vi "Main_11a.vi"() -> ()   [LabVIEW 2020]
uses:
  4985a7b0-beb7-44e5-b21a-1b7cc2dea417.vi
  <vilib>/Comparison/Less/Less Functor/Less Functor.lvclass
panel:
  out "Post Round":T1(array[cluster])
  out "Answer":i32
  in  "Puzzle":string="Monkey 0:\n  Starting items: 72, 97\n  Operation: new = old * 13\n  Test: divisible by 19\n    If true: throw to monkey 5\n    If false: throw to monkey 6\n\nMonkey 1:\n  Starting items: 55, 70, 90, 74, 95\n  Operation: new = old * old\n  Test: divisible by 7\n    If true: throw to monkey 5\n    If false: throw to monkey 0\n\nMonkey 2:\n  Starting items: 74, 97, 66, 57\n  Operation: new = old + 6\n  Test: divisible by 17\n    If true: throw to monkey 1\n    If false: throw to monkey 0\n\nMonkey 3:\n  Starting items: 86, 54, 53\n  Operation: new = old + 2\n  Test: divisible by 13\n    If true: throw to monkey 1\n    If false: throw to monkey 2\n\nMonkey 4:\n  Starting items: 50, 65, 78, 50, 62, 99\n  Operation: new = old + 3\n  Test: divisible by 11\n    If true: throw to monkey 3\n    If false: throw to monkey 7\n\nMonkey 5:\n  Starting items: 90\n  Operation: new = old + 4\n  Test: divisible by 2\n    If true: throw to monkey 4\n    If false: throw to monkey 6\n\nMonkey 6:\n  Starting items: 88, 92, 63, 94, 96, 82, 53, 53\n  Operation: new = old + 8\n  Test: divisible by 5\n    If true: throw to monkey 4\n    If false: throw to monkey 7\n\nMonkey 7:\n  Starting items: 70, 60, 71, 69, 77, 70, 98\n  Operation: new = old * 7\n  Test: divisible by 3\n    If true: throw to monkey 2\n    If false: throw to monkey 3"
  in  "Example":string="Monkey 0:\n  Starting items: 79, 98\n  Operation: new = old * 19\n  Test: divisible by 23\n    If true: throw to monkey 2\n    If false: throw to monkey 3\n\nMonkey 1:\n  Starting items: 54, 65, 75, 74\n  Operation: new = old + 6\n  Test: divisible by 19\n    If true: throw to monkey 2\n    If false: throw to monkey 0\n\nMonkey 2:\n  Starting items: 79, 60, 97\n  Operation: new = old * old\n  Test: divisible by 13\n    If true: throw to monkey 1\n    If false: throw to monkey 3\n\nMonkey 3:\n  Starting items: 74\n  Operation: new = old + 3\n  Test: divisible by 17\n    If true: throw to monkey 0\n    If false: throw to monkey 1"
  # "58056"
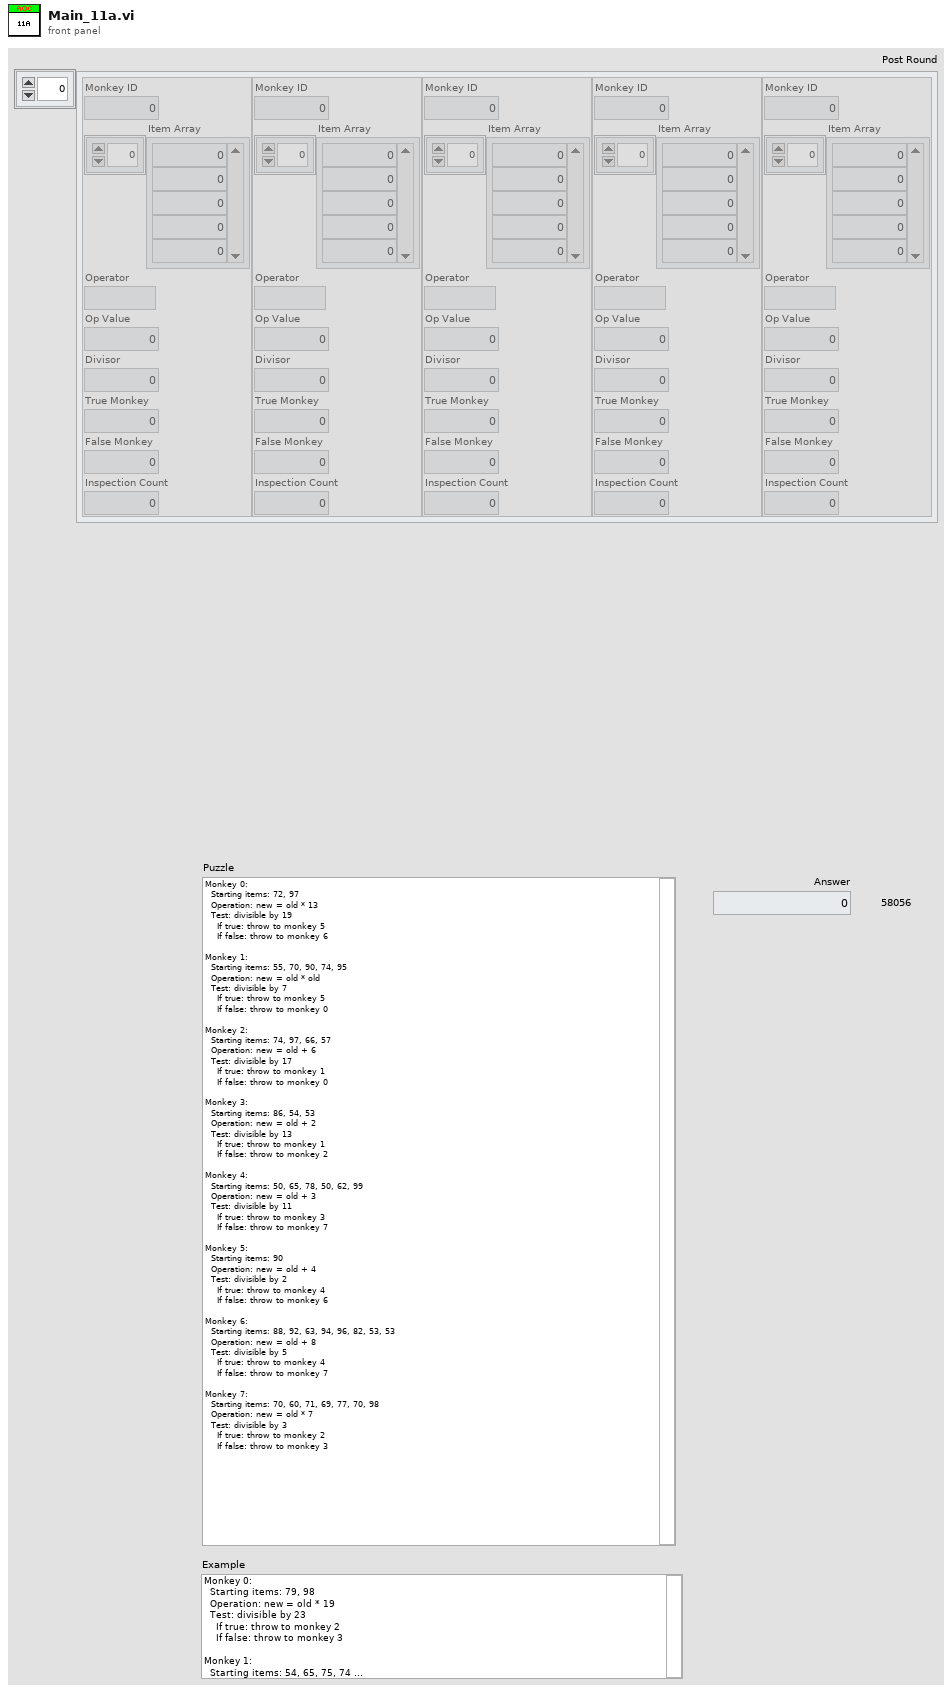
[diagram p1: front panel]
types:
  T1 = cluster{"Monkey ID":i32, "Item Array":i32[], "Operator":string, "Op Value":i32, "Divisor":i32, "True Monkey":i32, "False Monkey":i32, "Inspection Count":i32}[]
  T2 = cluster{"Monkey ID":i32, "Item Array":i32[], "Operator":string, "Op Value":i32, "Divisor":i32, "True Monkey":i32, "False Monkey":i32, "Inspection Count":i32}
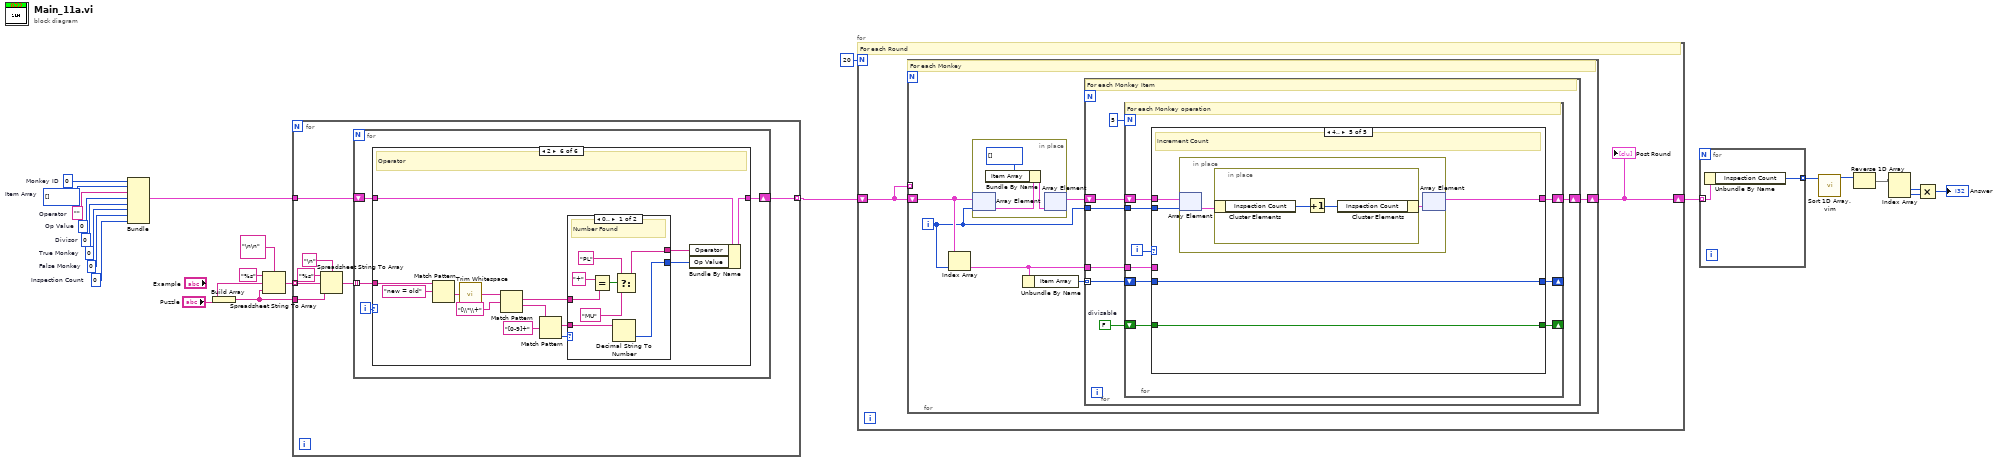
[diagram p0: block diagram]
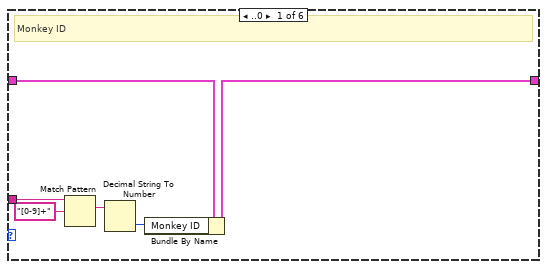
[diagram p2: hidden frame]
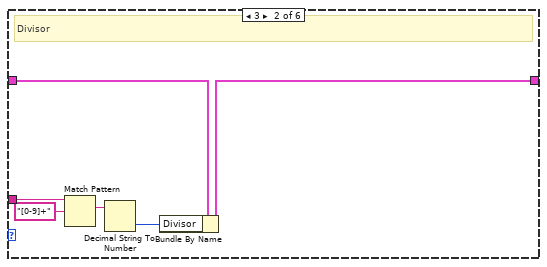
[diagram p3: hidden frame]
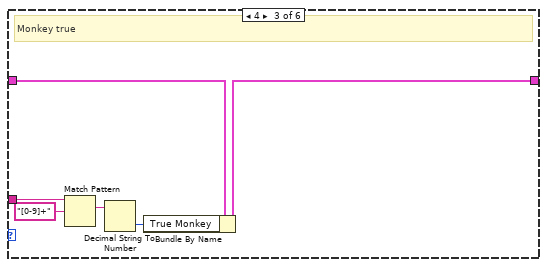
[diagram p4: hidden frame]
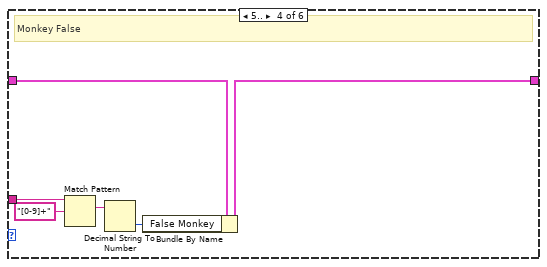
[diagram p5: hidden frame]
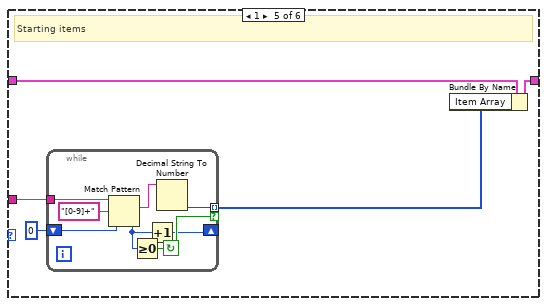
[diagram p6: hidden frame]
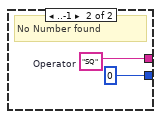
[diagram p7: hidden frame]
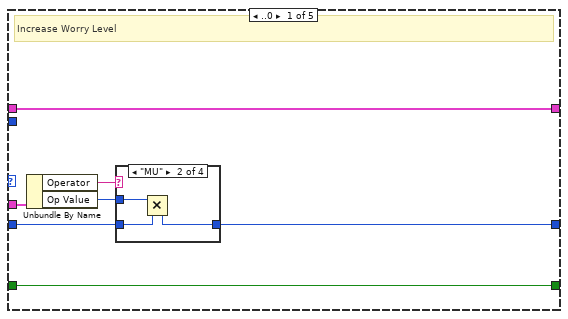
[diagram p8: hidden frame]
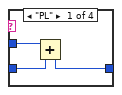
[diagram p9: hidden frame]
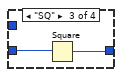
[diagram p10: hidden frame]
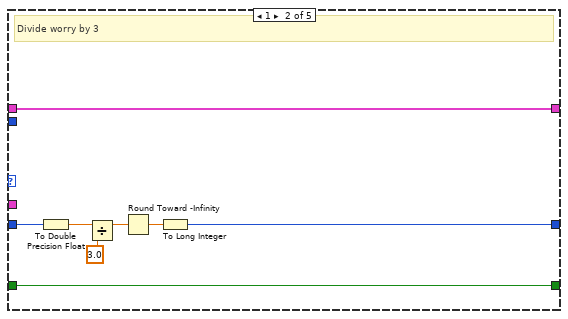
[diagram p12: hidden frame]
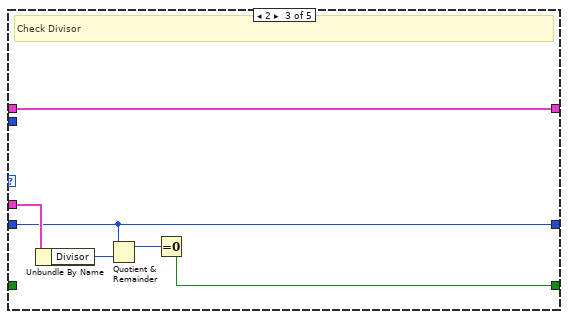
[diagram p13: hidden frame]
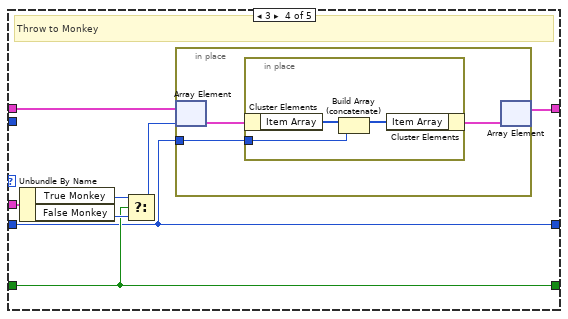
[diagram p14: hidden frame]
diagram:
  w9 = 0  # Inspection Count
  w12 = 0  # False Monkey
  w13 = 0  # True Monkey
  w14 = 0  # Divisor
  w15 = 0  # Op Value
  w16 = ""  # Operator
  w17 = i32[] []  # Item Array
  w18 = 0  # Monkey ID
  n1 = Bundle("Monkey ID"=w18, "Item Array"=w17, "Operator"=w16, "Op Value"=w15, "Divisor"=w14, "True Monkey"=w13, "False Monkey"=w12, "Inspection Count"=w9) -> (w11:T2)  [unwired: 1 in]
  n2 = Build Array("Puzzle") -> (w19:string[])
  n3 = Spreadsheet String To Array(delimiter (Tab)="\n\n", format string="%s", spreadsheet string="Puzzle", array type (2D Dbl)=w19) -> (array=w20:string[])
  n4 = for {
    tunnel: w20 -> [w30] mode=indexing
    tunnel: w19 -> [w27]
    tunnel: w11 -> [w25]
    tunnel: [w24] -> w10 mode=indexing
    n5 = Spreadsheet String To Array(delimiter (Tab)="\n", format string="%s", spreadsheet string=w30, array type (2D Dbl)=w27) -> (array=w26:string[])
    n6 = for {
      tunnel: w26 -> [w31] mode=indexing
      shift-right: [w32] -> w24
      shift-left: w25 -> [w33]
      i -> [w34]
      n7 = case shown="2" w34 {
        tunnel: w33 -> [w40 w46 w52 w58 w63 w85]
        tunnel: [w39 w45 w51 w57 w62 w84] -> w32
        tunnel: w31 -> [w38 w44 w50 w56 w61 w83]
        frame ..0 {
          # "Monkey ID"
          n8 = Match Pattern(string=w38, regular expression="[0-9]+") -> (match substring=w36:string)  [unwired: 1 in, 3 out]
          n9 = Decimal String To Number(string=w36) -> (number=w35:i32)  [unwired: 2 in, 1 out]
          n10 = Bundle By Name(cluster=w40, "Monkey ID"=w35) -> (w39:T2)
        }
        frame 3 {
          # "Divisor"
          n11 = Match Pattern(string=w44, regular expression="[0-9]+") -> (match substring=w42:string)  [unwired: 1 in, 3 out]
          n12 = Decimal String To Number(string=w42) -> (number=w41:i32)  [unwired: 2 in, 1 out]
          n13 = Bundle By Name(cluster=w46, "Divisor"=w41) -> (w45:T2)
        }
        frame 4 {
          # "Monkey true"
          n14 = Match Pattern(string=w50, regular expression="[0-9]+") -> (match substring=w48:string)  [unwired: 1 in, 3 out]
          n15 = Decimal String To Number(string=w48) -> (number=w47:i32)  [unwired: 2 in, 1 out]
          n16 = Bundle By Name(cluster=w52, "True Monkey"=w47) -> (w51:T2)
        }
        frame 5.. {
          # "Monkey False"
          n17 = Match Pattern(string=w56, regular expression="[0-9]+") -> (match substring=w54:string)  [unwired: 1 in, 3 out]
          n18 = Decimal String To Number(string=w54) -> (number=w53:i32)  [unwired: 2 in, 1 out]
          n19 = Bundle By Name(cluster=w58, "False Monkey"=w53) -> (w57:T2)
        }
        frame 1 {
          # "Starting items"
          n20 = while {
            tunnel: w61 -> [w71]
            tunnel: [w67] -> w60 mode=indexing if=w69
            shift-right: [w65] -> _
            shift-left: 0 -> [w64]
            stop <- w69 continue-if-true
            n21 = Match Pattern(string=w71, regular expression="[0-9]+", offset (0)=w64) -> (match substring=w68:string, offset past match=w66:i32)  [unwired: 2 out]
            n22 = Greater Or Equal To 0?(x=w66) -> (x >= 0?=w69:bool)
            n23 = Increment(x=w66) -> (x+1=w65:i32)
            n24 = Decimal String To Number(string=w68) -> (number=w67:i32)  [unwired: 2 in, 1 out]
          }
          n25 = Bundle By Name(cluster=w63, "Item Array"=w60) -> (w62:T2)
        }
        frame 2 {
          # "Operator"
          n26 = Match Pattern(string=w83, regular expression="new = old") -> (after substring=w81:string)  [unwired: 1 in, 3 out]
          n27 = call <vilib>:"Trim Whitespace.vi"("string"=w81) -> ("trimmed string"=w79:string)  [unwired: 1 in]
          n28 = Match Pattern(string=w79, regular expression="[\\*\\+") -> (match substring=w73:string, after substring=w78:string)  [unwired: 1 in, 2 out]
          n29 = Match Pattern(string=w78, regular expression="[0-9]+") -> (match substring=w72:string, offset past match=w76:i32)  [unwired: 1 in, 2 out]
          n30 = case shown="0.." w76 {
            tunnel: [w88 w95] -> w75
            tunnel: [w86 0] -> w74
            tunnel: w73 -> [w92 _]
            tunnel: w72 -> [w87 _]
            frame 0.. {
              # "Number Found"
              n31 = Equal?(x="+", y=w92) -> (x = y?=w91:bool)
              n32 = Decimal String To Number(string=w87) -> (number=w86:i32)  [unwired: 2 in, 1 out]
              n33 = Select(t="PL", s=w91, f="MU") -> (s? t:f=w88:string)
            }
            frame ..-1 {
              w95 = "SQ"  # Operator
              # "No Number found"
            }
          }
          n34 = Bundle By Name(cluster=w85, "Operator"=w75, "Op Value"=w74) -> (w84:T2)
        }
      }
    }
  }
  n35 = for {
    N: 20 -> [_]
    shift-right: [w96] -> w8
    shift-left: w10 -> [w97]
    # "For each Round"
    n36 = for {
      shift-right: [w103] -> w96
      shift-left: w97 -> [w100]
      tunnel: w97 -> [_] mode=indexing
      i -> [w99]
      # "For each Monkey"
      n37 = Index Array(array=w100, index=w99) -> (element=w98:T2)
      n38 = in-place {
        n39 = in-place-array #1(w100, w99) -> (w106:T2)
        n40 = Bundle By Name(cluster=w106, "Item Array"=i32[] []) -> (w105:T2)
        n41 = in-place-array #1(w105) -> (w101:T1)  [unwired: 1 out]
      }
      n42 = Unbundle By Name(w98) -> ("Item Array"=w102:i32[])
      n43 = for {
        tunnel: w98 -> [w111]
        tunnel: w102 -> [w112] mode=indexing
        shift-right: [w107] -> w103
        shift-left: w101 -> [w110]
        tunnel: w99 -> [w108]
        w109 = FALSE  # divisable
        # "For each Monkey Item"
        n44 = for {
          N: 5 -> [_]
          shift-right: [w118] -> _
          shift-left: w112 -> [w121]
          tunnel: w111 -> [w120]
          shift-right: [w117] -> w107
          shift-left: w110 -> [w119]
          shift-right: [w115] -> _
          shift-left: w109 -> [w116]
          tunnel: w108 -> [w114]
          i -> [w122]
          # "For each Monkey operation"
          n45 = case shown="4.." w122 {
            tunnel: w121 -> [w126 w146 w147 w153 w167]
            tunnel: w120 -> [w129 _ w151 w160 _]
            tunnel: w119 -> [w124 w140 w152 w156 w170]
            tunnel: [w125 w141 w147 w153 w167] -> w118
            tunnel: [w124 w140 w152 w155 w169] -> w117
            tunnel: w116 -> [w123 w139 _ w157 w171]
            tunnel: [w123 w139 w148 w157 w171] -> w115
            tunnel: w114 -> [_ _ _ _ w168]
            frame ..0 {
              # "Increase Worry Level"
              n46 = Unbundle By Name(w129) -> ("Operator"=w128:string, "Op Value"=w127:i32)
              n47 = case shown="\"MU\"" w128 {
                tunnel: w127 -> [w132 w135 _ _]
                tunnel: w126 -> [w131 w134 w137 w138]
                tunnel: [w130 w133 w136 w138] -> w125
                frame "PL" {
                  n48 = Add(x=w132, y=w131) -> (x+y=w130:i32)
                }
                frame "MU" {
                  n49 = Multiply(x=w135, y=w134) -> (x*y=w133:i32)
                }
                frame "SQ" {
                  n50 = Square(x=w137) -> (x^2=w136:i32)
                }
                frame Default {
                }
              }
            }
            frame 1 {
              # "Divide worry by 3"
              n51 = To Double Precision Float(number=w146) -> (double precision float=w145:dbl)
              n52 = Divide(x=w145, y=3.0) -> (x/y=w143:dbl)
              n53 = Round Toward -Infinity(1:w143) -> (0:w142:dbl)
              n54 = To Long Integer(number=w142) -> (32bit integer=w141:i32)
            }
            frame 2 {
              # "Check Divisor"
              n55 = Unbundle By Name(w151) -> ("Divisor"=w150:i32)
              n56 = Quotient & Remainder(x=w147, y=w150) -> (x-y*floor(x/y)=w149:i32)  [unwired: 1 out]
              n57 = Equal To 0?(x=w149) -> (x = 0?=w148:bool)
            }
            frame 3 {
              # "Throw to Monkey"
              n58 = Unbundle By Name(w160) -> ("True Monkey"=w159:i32, "False Monkey"=w158:i32)
              n59 = Select(t=w159, s=w157, f=w158) -> (s? t:f=w154:i32)
              n60 = in-place {
                in-place-border: w153 -> [w161]
                n61 = in-place-array #2(w156, w154) -> (w163:T2)
                n62 = in-place {
                  in-place-border: w161 -> [w165]
                  n63 = in-place-cluster #3(w163) -> ("Item Array"=w166:i32[])
                  n64 = Build Array (concatenate)(w166, w165) -> (w164:i32[])
                  n65 = in-place-cluster #3("Item Array"=w164) -> (w162:T2)
                }
                n66 = in-place-array #2(w162) -> (w155:T1)  [unwired: 1 out]
              }
            }
            frame 4.. {
              # "Increment Count"
              n67 = in-place {
                n68 = in-place-array #4(w170, w168) -> (w173:T2)
                n69 = in-place {
                  n70 = in-place-cluster #5(w173) -> ("Inspection Count"=w175:i32)
                  n71 = Increment(x=w175) -> (x+1=w174:i32)
                  n72 = in-place-cluster #5("Inspection Count"=w174) -> (w172:T2)
                }
                n73 = in-place-array #4(w172) -> (w169:T1)  [unwired: 1 out]
              }
            }
          }
        }
      }
    }
    "Post Round" <- w96
  }
  n74 = for {
    tunnel: w8 -> [w177] mode=indexing
    tunnel: [w176] -> w7 mode=indexing
    n75 = Unbundle By Name(w177) -> ("Inspection Count"=w176:i32)
  }
  n76 = call "Sort 1D Array.vim"("unsorted array"=w7) -> ("sorted array"=w6:i32[])  [unwired: 10 in]
  n77 = Reverse 1D Array(array=w6) -> (reversed array=w5:i32[])
  n78 = Index Array(array=w5) -> (element #1=w3:i32, element #2=w4:i32)  [unwired: 2 in]
  n79 = Multiply(x=w3, y=w4) -> (x*y=→"Answer":i32)
